vi "Joystick Close to zeroed.vi"(11 "Joystick":dbl) -> (3 "=0?":bool)   [LabVIEW 2018]
panel:
  in  "Deadband":dbl=0.06
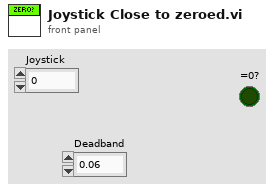
[diagram p1: front panel]
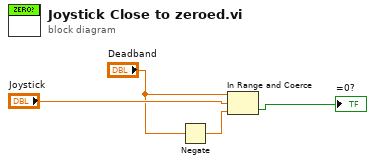
[diagram p0: block diagram]
diagram:
  n1 = Negate(x="Deadband") -> (-x=w3:dbl)
  n2 = In Range and Coerce(upper limit="Deadband", x="Joystick", lower limit=w3) -> (In Range?=→"=0?":bool)  [unwired: 1 out]
